vi "Generalized Eigenvalues and Vectors.vi"   [LabVIEW 2024, in "NI_AALPro.lvlib"]
doc: "<p>Computes the generalized right eigenvalues and eigenvectors of the matrix pair <strong>A</strong> and <strong>B</strong>. The data types you wire to the <strong>A</strong> and <strong>B</strong> inputs determine the polymorphic instance to use.</p>"
uses:
  NI_AALPro.lvlib
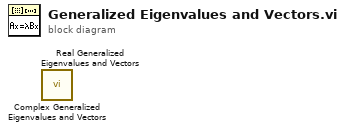
[diagram p0: block diagram]
diagram:
  n1 = call "Complex Generalized Eigenvalues and Vectors.vi"() -> ()  [unwired: 6 in, 3 out]
  n2 = call "Real Generalized Eigenvalues and Vectors.vi"() -> ()  [unwired: 6 in, 3 out]
